vi "Draw.vi"(8 "error in (no error)":errorcluster, 10 "2D Picture in":picture, 11 "UMLClass in":refnum<class "UMLClass.lvclass">) -> (0 "error out":errorcluster, 2 "2D Picture out":picture, 3 "UMLClass out":refnum<class "UMLClass.lvclass">)   [LabVIEW 2021, in "Picture2D.lvlib" / "UMLClass.lvclass"]
uses:
  UMLClass.lvclass
  C:/Users/Dany/OneDrive/LabVIEW/Class/Picture2D/Shape/Shape.lvclass
  UMLClass.lvclass/UMLClass.ctl
  GetClassName.vi
  GetProperties.vi
  GetMethods.vi
  Shape/Shape.lvclass
  Color/Color.lvclass
  Point/Point.lvclass
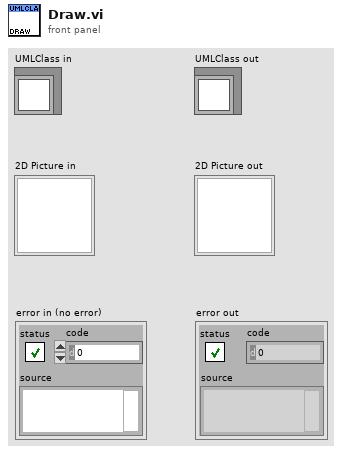
[diagram p1: front panel]
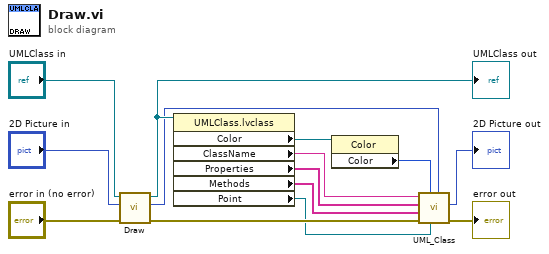
[diagram p0: block diagram]
diagram:
  n1 = call-parent "Draw.vi"("error in (no error)"="error in (no error)", "2D Picture in"="2D Picture in", "Shape in"="UMLClass in") -> ("error out"=w3:errorcluster, "2D Picture out"=w7:picture, "Shape out"=w11:refnum<class "UMLClass.lvclass">)  [unwired: 6 in]
  "UMLClass out" <- w11
  n2 = property class="UMLClass.lvclass"(reference=w11) -> ("Color"=w5:refnum<class "Color.lvclass">, "ClassName"=w10:string, "Properties"=w9:string[], "Methods"=w8:string[], "Point"=w1:refnum<class "Point.lvclass">)  [unwired: 1 in, 2 out]
  n3 = property class="Color"(reference=w5) -> ("Color"=w4:u32)  [unwired: 1 in, 2 out]
  n4 = call "UML_Class.vi"("2D Picture in"=w7, "Point"=w1, "Color"=w4, "error in (no error)"=w3, "Methods"=w8, "Properties"=w9, "Class Name"=w10) -> ("error out"=→"error out":errorcluster, "2D Picture out"=→"2D Picture out":picture)  [unwired: 2 in, 1 out]
